vi "Measure Current.vi"(6 "Result Multiplier":dbl=1000000.0 format="%#_13e", 7 "Channel Lists":string[](array[string]), 8 "error in (no error)":errorcluster, 10 "Delay Time (s)":dbl, 11 "DCPower Sessions In":refnum<k15>[](array[refnum])) -> (0 "error out":errorcluster, 1 "current measurements":dbl[][](array[numeric]), 3 "DCPower Sessions Out":refnum<k15>[](array[refnum]))   [LabVIEW 2013]
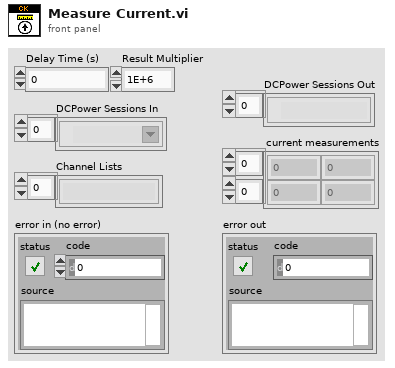
[diagram p1: front panel]
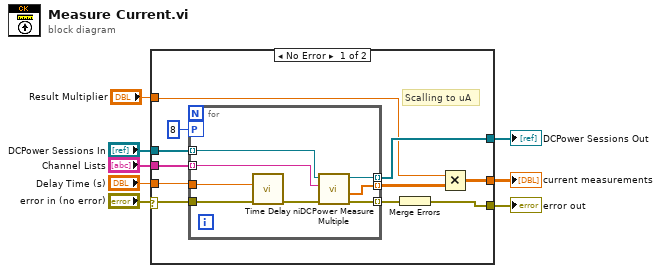
[diagram p0: block diagram]
diagram:
  n1 = case shown="No Error" "error in (no error)" {
    selector: "error in (no error)" -> [w11 w28]
    tunnel: "Channel Lists" -> [w19 _]
    tunnel: "DCPower Sessions In" -> [w18 w29]
    tunnel: [w17 w29] -> w6
    tunnel: [w15 w28] -> w5
    tunnel: "Delay Time (s)" -> [w14 _]
    tunnel: [w12 _] -> w3
    tunnel: "Result Multiplier" -> [w9 _]
    frame No Error {
      # "Scalling to uA"
      n2 = for {
        tunnel: w11 -> [w23]
        tunnel: w18 -> [w21] mode=indexing
        tunnel: w19 -> [w25] mode=indexing
        tunnel: [w27] -> w16 mode=indexing
        tunnel: [w26] -> w13 mode=indexing
        tunnel: [w24] -> w17 mode=indexing
        tunnel: w14 -> [w20]
        workers-P: 8 -> [_]
        n3 = call "Time Delay"("error in (no error)"=w23, "Delay Time (s)"=w20) -> ("error out"=w22:errorcluster)  [unwired: 9 in]
        n4 = call <instrlib>:"niDCPower Measure Multiple.vi"("error in (no error)"=w22, "channel name"=w25, "instrument handle"=w21) -> ("error out"=w27:errorcluster, "current measurements"=w26:dbl[], "instrument handle out"=w24:refnum<k15>)  [unwired: 5 in, 1 out]
      }
      n5 = Merge Errors(w16) -> (w15:errorcluster)
      n6 = Multiply(x=w9, y=w13) -> (x*y=w12:dbl[][])
    }
    frame Error {
    }
  }
  "current measurements" <- w3
  "DCPower Sessions Out" <- w6
  "error out" <- w5
